vi "inicializacion_lora_sin_ok.vi"(11 "Direccion":i16=1 min=1 max=127 step=1) -> (3 "concatenated string 2":string)   [LabVIEW 2022 SP3]
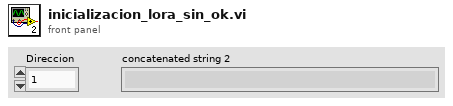
[diagram p1: front panel]
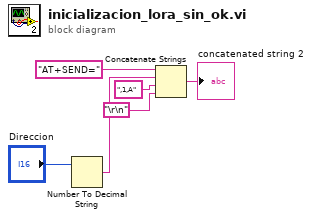
[diagram p0: block diagram]
diagram:
  n1 = Number To Decimal String(number="Direccion") -> (decimal integer string=w6:string)  [unwired: 1 in]
  n2 = Concatenate Strings("AT+SEND=" ("string"), w6, ",1,A" ("string"), "\r\n") -> (→"concatenated string 2":string)
